vi "IC measurment N6972A - Published.vi"() -> ()   [LabVIEW 2022 SP3]
doc: "This example demonstrates how to configure a list in current priority mode."
uses:
  <vilib>/Analysis/baseanly.llb/Mean (DBL).vi
  <instrlib>/Agilent 34420/Public/Data/Read (Multiple Points).vi
  <instrlib>/Agilent N6900 N7900 Series/Agilent N6900 N7900 Series.lvlib
  <instrlib>/Agilent 34420/Agilent 34420.lvlib
  <vilib>/Analysis/NI_AALBase.lvlib
  <vilib>/Utility/TDMS File Viewer/NI_TDMS File Viewer.lvlib
panel:
  out "Boolean":bool
  out "String":string="WARNING: FILE PATH EXISTS"
  in  "Path":path=path "C:/Users/kumarr3/OneDrive - Victoria University of Wellington - STAFF/Documents/DataFiles/NoLoad" caption="Load File Path or Directory"
  in  "Conduct Experiment\n\n\nLoad Experiment":bool
  in  "relative path (file or folder)":path=path "Test.tdms"
  in  "base path":path=path "C:/Users/kumarr3/OneDrive - Victoria University of Wellington - STAFF/Documents/DataFiles"
  in  "Tab Control":T1(tab)
  in  "N6972A VISA resource name":refnum<visa-resource-name>="USB0::0x0957::0x3407::MY63000447::INSTR"
  in  "Current Priority Voltage Limit":dbl=1.0
  in  "34420A VISA resource name":refnum<visa-resource-name>="COM3"
  in  "Resolution (1E-9)":dbl=1e-09
  in  "Manual Range (0.001)":dbl=0.001
  in  "Auto Range (T: Enable)":bool=TRUE
  in  "Serial Configuration":T2={"Baud Rate"=9600, "Parity"=0, "Data Bits"=8} {"Data Bits" items=["7"=7, "8"=8]; "Parity" items=["None", "Odd", "Even", "Mark", "Space"]; "Baud Rate" items=["300"=300, "600"=600, "1200"=1200, "2400"=2400, "4800"=4800, "9600"=9600]}
  in  "Function (0: DC Volts)":u16(ring) items=["DC Volts", "DC Voltage Ratio", "DC Voltage Difference", "2 Wire Resistance", "4 Wire Resistance", "Temperature"]
  in  "Channel (1: Channel 1)":u16(ring)=1 items=["Channel 1"=1, "Channel 2"=2]
  in  "Filter On/Off":string(combo)
  in  "Voltmeter Offset Sample Count":i32=10
  in  "Integration Time (4: 10 NPLCs)":u16(ring)=4 items=["0.02 NPLC", "0.2 NPLC", "1 NPLC", "2 NPLCs", "10 NPLCs", "20 NPLCs", "100 NPLCs", "200 NPLCs"]
  out "Waveform Chart":dbl(graph)
  in  "Measure Temperature?":bool
  out "Temperature Chart":dbl[](graph)=[25.735546538805686]
  out "?":string
  out "Progress Bar":dbl(slide) scale=0.0..1000.0
  in  "Minutes  / Seconds":bool
  in  "Hours / Minutes":bool
  out "Current Run":i32
  out "Number of Measurements":dbl
  in  "RUN MULTIPLE MEASUREMENTS":bool
  in  "Measurement Interval":dbl
  in  "Total Measurement Time":dbl
  out "XY Graph":cluster{dbl[], dbl[]}(graph)
  out "RMS Current":dbl
  out "uV/cm":dbl
  out "Voltmeter offset (µV)":dbl format="%e"
  out "Current array":dbl[](array[numeric])
  out "Voltage  array":dbl[](array[numeric])
  out "?":bool
  in  "Volt. Tap threshold (uV/cm)":dbl=0.25 format="%.2f"
  in  "Current increment above µV threshold [A]":dbl=0.1 format="%.2f"
  out "?":bool
  in  "Current increment 2 [A]":dbl=0.2 format="%.2f"
  in  "Current limit 1 [A]":dbl=38.0 format="%.2f"
  in  "Initial Current increment  [A]":dbl=5.0 format="%.2f"
  out "Max volt. reached":bool
  out "Max. current reached":bool
  in  "Max. Volt. Tap Voltage (uV/cm)":dbl=10.0
  in  "Maximum current (A)":dbl=48.0
  in  "Volt. Tap Distance (cm)":dbl=1.6
  in  "stop":bool
  out "Calibrating Offset?":bool
  out "Offset V vals":dbl[](array[numeric])
  out "Waiting Time Elapsed":i32 format="%<%H:%M:%S%2u>t"
  out "Start Time":timestamp
  out "Terminated Temp Msre":bool=TRUE
  in  "Temperature Reading Iterval(s)":u32=1
  in  "Ramp interval (s)":u32
  out "median Ic":dbl format="%0.2f"
  out "Current Run":cluster{dbl[], dbl[]}(graph) caption="XY Graph"
  out "Historial Results":cluster{dbl[], dbl[]}[](graph) caption="XY Graph"
  out "Ic Array":dbl[](array[numeric])
  out "n Array":dbl[](array[numeric])
  out "n Values Graph":dbl[](graph)
  out "mean Ic":dbl format="%0.2f"
  out "mean n":dbl format="%0.2f"
  out "Ic Values Graph":dbl[](graph)
  out "median n":dbl format="%0.2f"
  out "Errors?":string[](array[string])
  out "XY Graph 2":cluster{timestamp[], dbl[]}(graph)
  out "median n":dbl format="%0.2f"
  out "n Values Graph":cluster{timestamp[], dbl[]}(graph)
  out "Ic Values Graph":cluster{timestamp[], dbl[]}(graph)
  out "n Array":dbl[](array[numeric])
  out "Ic Array":dbl[](array[numeric])
  out "mean n":dbl format="%0.2f"
  out "mean Ic (A)":dbl format="%0.2f"
  out "Historical Data":cluster{"Array":dbl[], "Array":dbl[]}[](graph)
  out "Number of Runs":dbl
  out "Experiment Description":variant
  out "median Ic (A)":dbl format="%0.2f"
  out "current time":timestamp
  # "Ic Test Controls"
  # "Experiment Control"
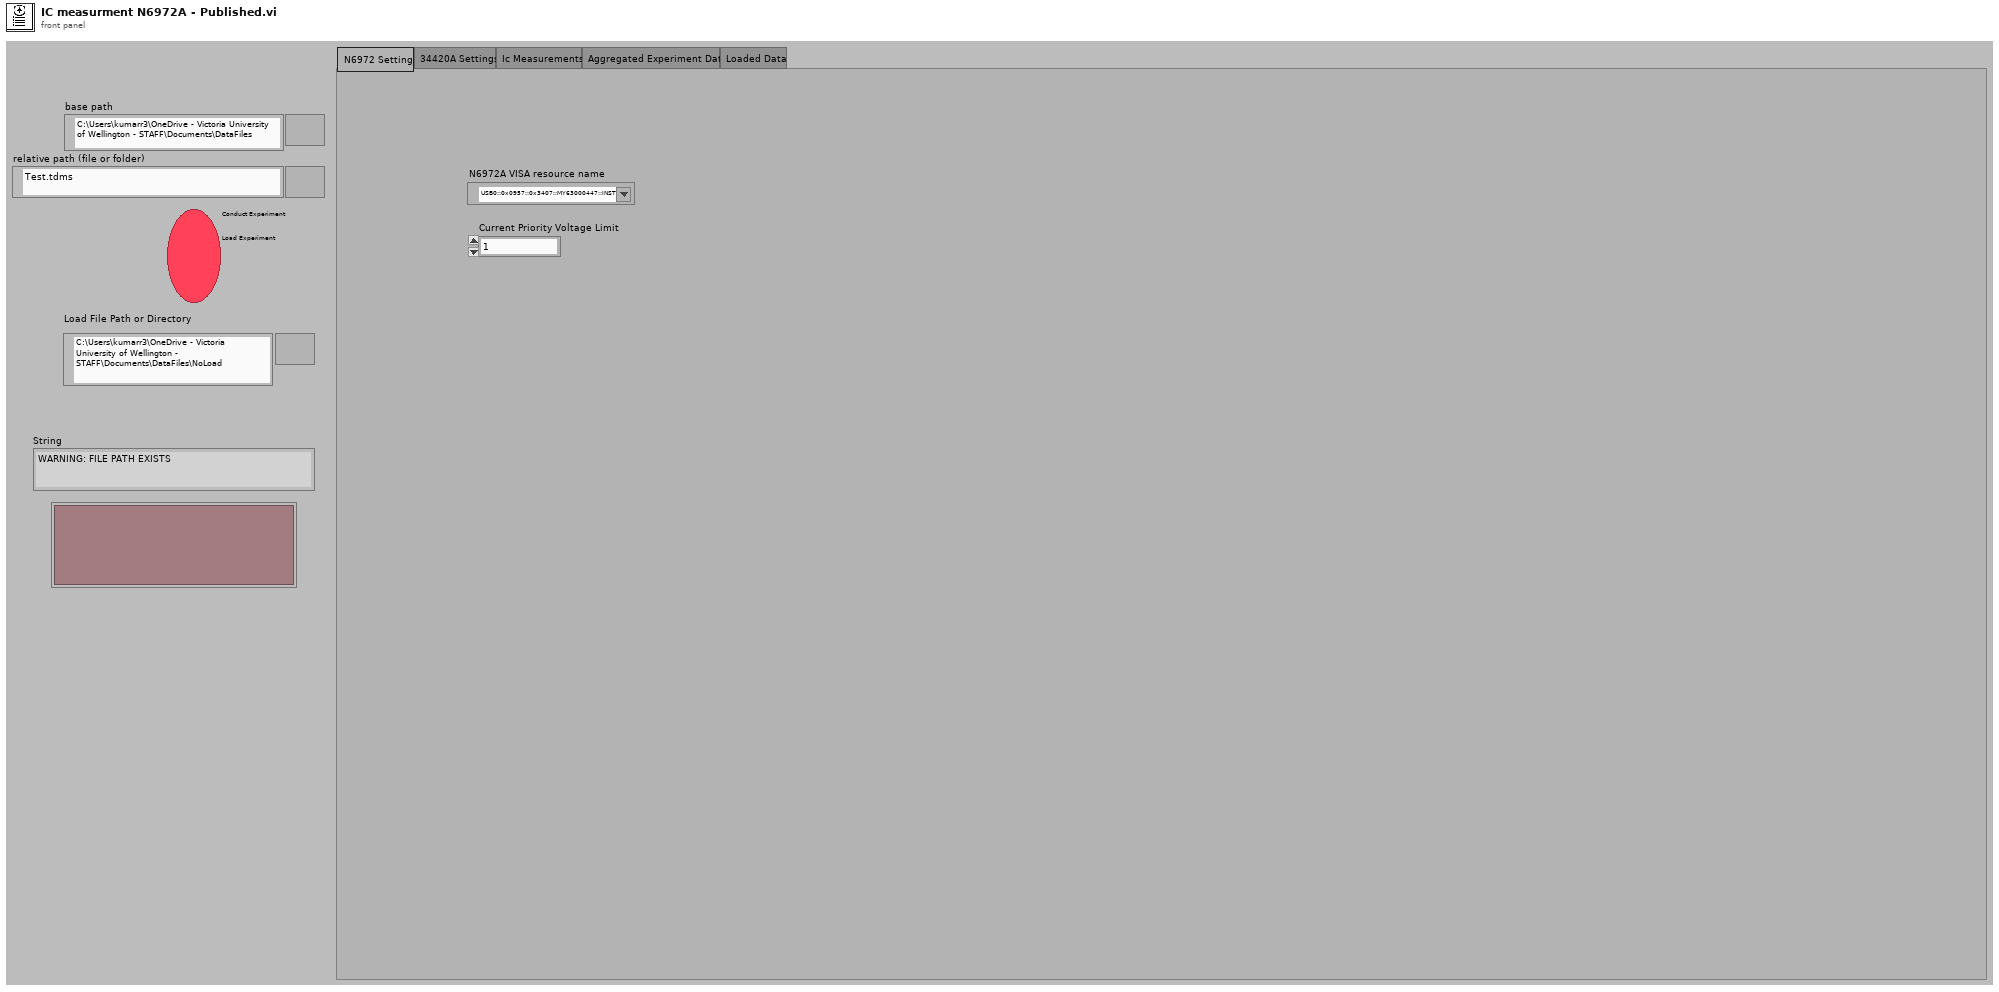
[diagram p1: front panel]
types:
  T1 = enum32{"N6972 Settings", "34420A Settings", "Ic Measurements", "Aggregated Experiment Data", "Loaded Data"}
  T2 = cluster{"Baud Rate":u32, "Parity":u16, "Data Bits":u16}
  T3 = enum16{"open", "open or create", "create or replace", "create", "open (read-only)"}
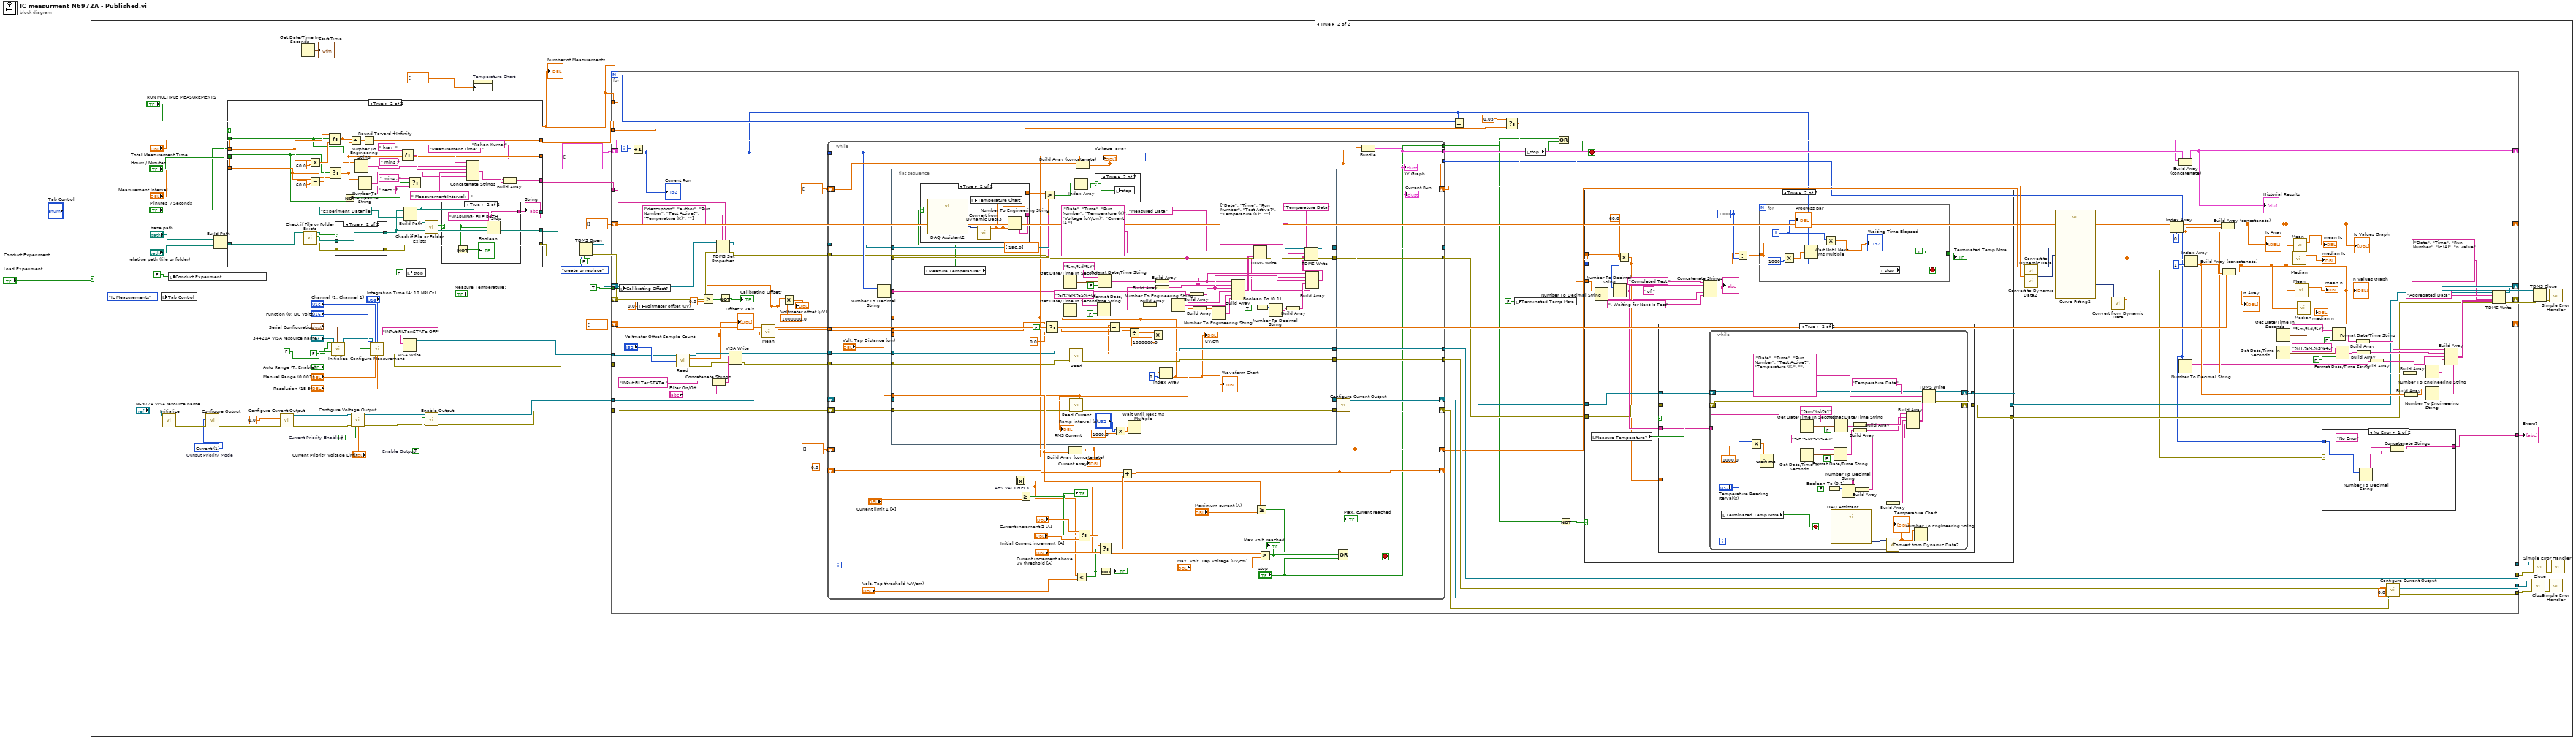
[diagram p0: block diagram]
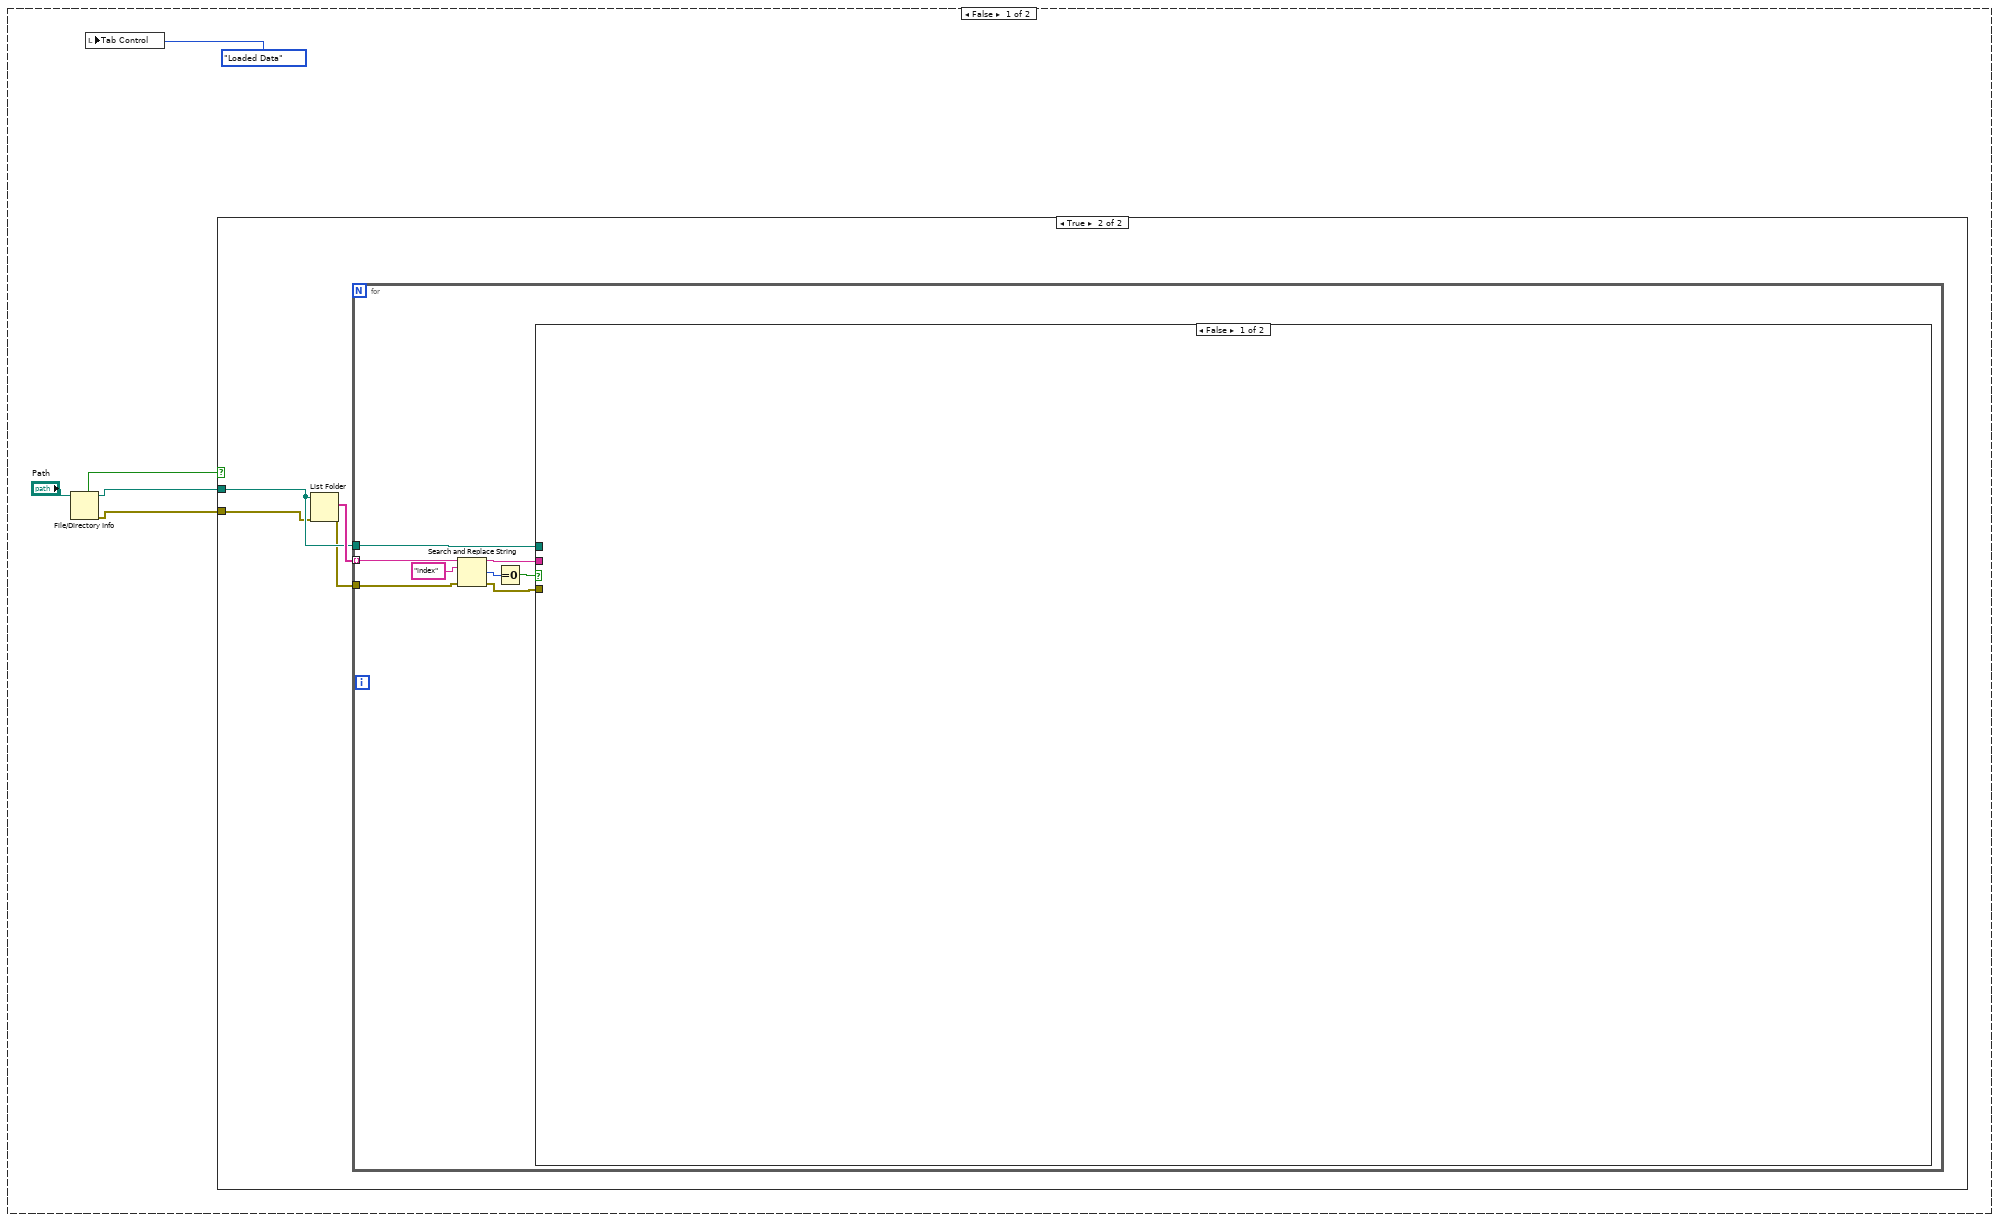
[diagram p2: hidden frame]
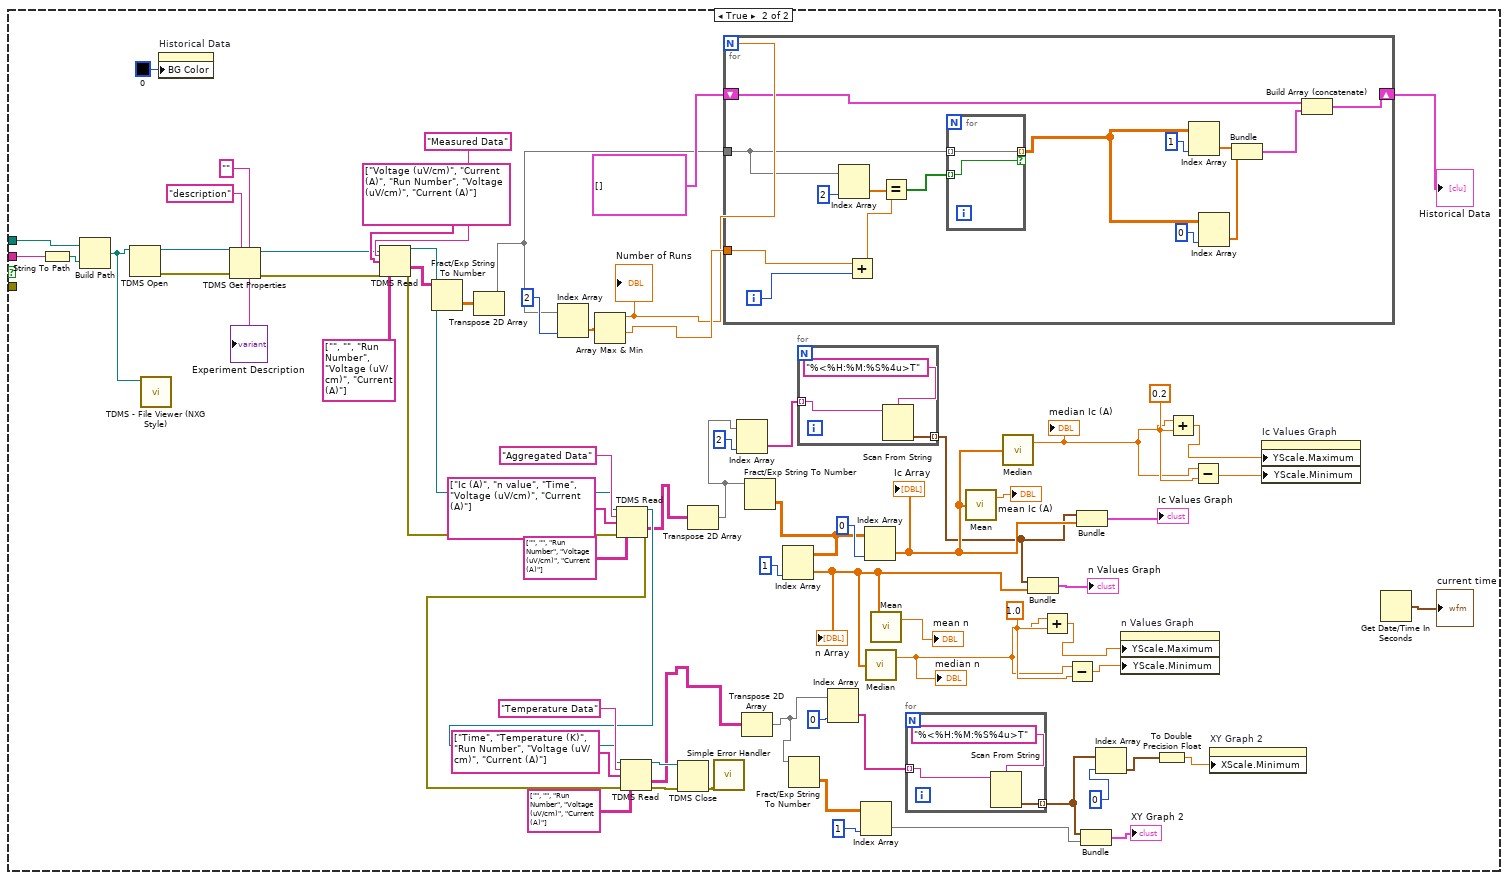
[diagram p4: hidden frame]
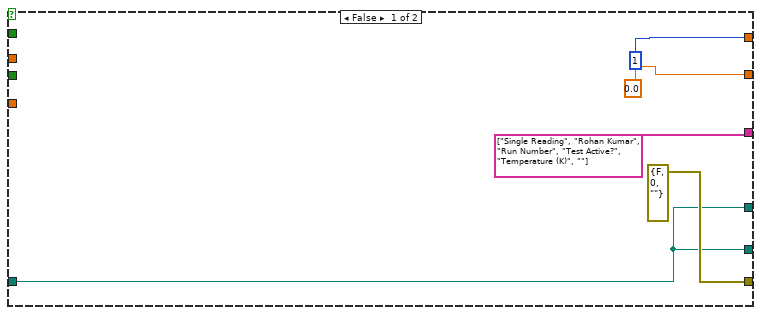
[diagram p5: hidden frame]
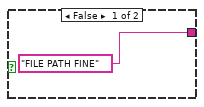
[diagram p6: hidden frame]
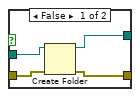
[diagram p7: hidden frame]
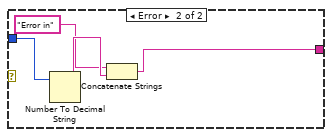
[diagram p8: hidden frame]
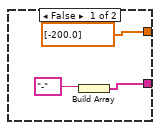
[diagram p12: hidden frame]
diagram:
  n1 = case shown="True" "Conduct Experiment\n\n\nLoad Experiment" {
    frame False {
      n2 = File/Directory Info(path="Path") -> (path out=w5:path, directory=w4:bool, error out=w3:errorcluster)  [unwired: 1 in, 4 out]
      n3 = local write "Tab Control"(T1."Loaded Data" ("Tab Control")) -> ()
      n4 = case shown="True" w4 {
        tunnel: w5 -> [_ w9]
        tunnel: w3 -> [_ w8]
        frame False {
        }
        frame True {
          n5 = List Folder(path=w9, error in=w8) -> (filenames=w10:string[], error out=w7:errorcluster)  [unwired: 2 in, 2 out]
          n6 = for {
            tunnel: w10 -> [w18] mode=indexing
            tunnel: w9 -> [w14]
            tunnel: w7 -> [w12]
            n7 = Search and Replace String(input string=w18, search string="index", error in=w12) -> (result string=w13:string, number of replacements=w16:i32, error out=w11:errorcluster)  [unwired: 5 in, 1 out]
            n8 = Equal To 0?(x=w16) -> (x = 0?=w15:bool)
            n9 = case shown="False" w15 {
              tunnel: w13 -> [_ w90]
              tunnel: w14 -> [_ w89]
              tunnel: w11 -> [_ _]
              frame False {
              }
              frame True {
                w27 = 1.0
                w29 = 0.2
                n10 = String To Path(string=w90) -> (path=w88:path)
                n11 = Build Path(base path=w89, name or relative path=w88) -> (appended path=w19:path)
                n12 = TDMS Open(11:w19) -> (0:w66:errorcluster, 3:w67:refnum<k34>)  [unwired: 6 in]
                n13 = call <vilib>:"TDMS - File Viewer (NXG Style).vi"("file in"=w19) -> ()  [unwired: 9 in, 2 out]
                n14 = property on="Historical Data" class="XYGraph (strict)"("BG Color"=u32 0 ("Plot Area:Colors:BG Color")) -> ()  [unwired: 2 in, 2 out]
                n15 = TDMS Get Properties(5:"", 7:"description", 8:w66, 11:w67) -> (0:w64:errorcluster, 3:w65:refnum<k34>, 4:→"Experiment Description":string)  [unwired: 2 in, 3 out]
                n16 = TDMS Read(0:w65, 5:"Measured Data" ("group name in"), 7:string[] ["Voltage (uV/cm)", "Current (A)", "Run Number", "Voltage (uV/cm)", "Current (A)"] ("channel name(s) in (Untitled)"), 11:w64, 12:string[][] [["", "", "Run Number", "Voltage (uV/cm)", "Current (A)"]] ("channel name(s) in (Untitled)")) -> (4:w54:refnum<k34>, 10:w84:string[][], 15:w53:errorcluster)  [unwired: 3 in, 3 out]
                n17 = Fract/Exp String To Number(string=w84) -> (number=w83:dbl[][])  [unwired: 3 in, 1 out]
                n18 = Transpose 2D Array(2D array=w83) -> (transposed array=w69:dbl[][])
                n19 = Index Array(array=w69, index (col)=2 ("disabled index (col)")) -> (element=w74:dbl[])  [unwired: 1 in]
                n20 = Array Max & Min(array=w74) -> (max value=w72:dbl, min value=w73:dbl)  [unwired: 2 out]
                "Number of Runs" <- w72
                n21 = TDMS Read(0:w54, 5:"Aggregated Data" ("group name in"), 7:string[] ["Ic (A)", "n value", "Time", "Voltage (uV/cm)", "Current (A)"] ("channel name(s) in (Untitled)"), 11:w53, 12:string[][] [["", "", "Run Number", "Voltage (uV/cm)", "Current (A)"]] ("channel name(s) in (Untitled)")) -> (4:w52:refnum<k34>, 10:w34:string[][], 15:w51:errorcluster)  [unwired: 3 in, 3 out]
                n22 = TDMS Read(0:w52, 5:"Temperature Data" ("group name in"), 7:string[] ["Time", "Temperature (K)", "Run Number", "Voltage (uV/cm)", "Current (A)"] ("channel name(s) in (Untitled)"), 11:w51, 12:string[][] [["", "", "Run Number", "Voltage (uV/cm)", "Current (A)"]] ("channel name(s) in (Untitled)")) -> (4:w56:refnum<k34>, 10:w48:string[][], 15:w55:errorcluster)  [unwired: 3 in, 3 out]
                n23 = TDMS Close(8:w55, 11:w56) -> (0:w60:errorcluster)  [unwired: 1 out]
                n24 = Transpose 2D Array(2D array=w34) -> (transposed array=w33:string[][])
                n25 = call <vilib>:"Simple Error Handler.vi"("error in (no error)"=w60) -> ()  [unwired: 2 in, 7 out]
                n26 = for {
                  N: w72 -> [_]
                  tunnel: w69 -> [w105]
                  tunnel: w73 -> [w103]
                  shift-right: [w97] -> w70
                  shift-left: cluster{dbl[], dbl[]}[] [] -> [w99]
                  i -> [w111]
                  n27 = Index Array(array=w105, index (col)=2 ("disabled index (col)")) -> (element=w106:dbl[])  [unwired: 1 in]
                  n28 = Add(x=w103, y=w111) -> (x+y=w104:dbl)
                  n29 = Equal?(x=w106, y=w104) -> (x = y?=w101:bool[])
                  n30 = for {
                    tunnel: w101 -> [w112] mode=indexing
                    tunnel: w105 -> [w113] mode=indexing
                    tunnel: [w113] -> w102 mode=indexing if=w112
                  }
                  n31 = Index Array(array=w102, index (col)=1 ("disabled index (col)")) -> (element=w108:dbl[])  [unwired: 1 in]
                  n32 = Index Array(array=w102, index (col)=0 ("disabled index (col)")) -> (element=w107:dbl[])  [unwired: 1 in]
                  n33 = Bundle(w108, w107) -> (w98:cluster{dbl[], dbl[]})  [unwired: 1 in]
                  n34 = Build Array (concatenate)(w99, w98) -> (w97:cluster{dbl[], dbl[]}[])
                }
                "Historical Data" <- w70
                n35 = Index Array(array=w33, index (col)=2 ("disabled index (col)")) -> (element=w40:string[])  [unwired: 1 in]
                n36 = Transpose 2D Array(2D array=w48) -> (transposed array=w45:string[][])
                n37 = Fract/Exp String To Number(string=w33) -> (number=w32:dbl[][])  [unwired: 3 in, 1 out]
                n38 = Index Array(array=w32, index (col)=1 ("disabled index (col)")) -> (element=w39:dbl[])  [unwired: 1 in]
                "n Array" <- w39
                n39 = Fract/Exp String To Number(string=w45) -> (number=w47:dbl[][])  [unwired: 3 in, 1 out]
                n40 = for {
                  tunnel: w40 -> [w93] mode=indexing
                  tunnel: [w91] -> w36 mode=indexing
                  n41 = Scan From String(format string="%<%H:%M:%S%4u>T" ("time format string (%c)"), input string=w93) -> (output 1=w91:timestamp)  [unwired: 3 in, 3 out]
                }
                n42 = Index Array(array=w45, index (col)=0 ("disabled index (col)")) -> (element=w44:string[])  [unwired: 1 in]
                n43 = Index Array(array=w47, index (col)=1 ("disabled index (col)")) -> (element=w43:dbl[])  [unwired: 1 in]
                n44 = Index Array(array=w32, index (col)=0 ("disabled index (col)")) -> (element=w37:dbl[])  [unwired: 1 in]
                "Ic Array" <- w37
                n45 = call <vilib>:"Median.vi"("X"=w39) -> ("median"=w24:dbl)  [unwired: 1 out]
                "median n" <- w24
                n46 = call-poly <vilib>:"Mean.vi"("X"=w39) -> ("mean"=→"mean n":dbl)  [unwired: 1 out]
                n47 = for {
                  tunnel: w44 -> [w96] mode=indexing
                  tunnel: [w94] -> w23 mode=indexing
                  n48 = Scan From String(format string="%<%H:%M:%S%4u>T" ("time format string (%c)"), input string=w96) -> (output 1=w94:timestamp)  [unwired: 3 in, 3 out]
                }
                n49 = call-poly <vilib>:"Mean.vi"("X"=w37) -> ("mean"=→"mean Ic (A)":dbl)  [unwired: 1 out]
                n50 = call <vilib>:"Median.vi"("X"=w37) -> ("median"=w28:dbl)  [unwired: 1 out]
                "median Ic (A)" <- w28
                n51 = Bundle(w36, w39) -> (→"n Values Graph":cluster{timestamp[], dbl[]})  [unwired: 1 in]
                n52 = Add(x=w24, y=w27) -> (x+y=w26:dbl)
                n53 = Subtract(x=w24, y=w27) -> (x-y=w25:dbl)
                n54 = Bundle(w36, w37) -> (→"Ic Values Graph":cluster{timestamp[], dbl[]})  [unwired: 1 in]
                n55 = Bundle(w23, w43) -> (→"XY Graph 2":cluster{timestamp[], dbl[]})  [unwired: 1 in]
                n56 = Index Array(array=w23, index=0 ("disabled index (col)")) -> (element=w21:timestamp)
                n57 = property on="n Values Graph" class="XYGraph (strict)"("YScale.Maximum"=w26, "YScale.Minimum"=w25) -> ()  [unwired: 2 in, 2 out]
                n58 = To Double Precision Float(number=w21) -> (double precision float=w20:dbl)
                n59 = Add(x=w28, y=w29) -> (x+y=w30:dbl)
                n60 = Subtract(x=w28, y=w29) -> (x-y=w31:dbl)
                n61 = property on="XY Graph 2" class="XYGraph (strict)"("XScale.Minimum"=w20) -> ()  [unwired: 2 in, 2 out]
                n62 = property on="Ic Values Graph" class="XYGraph (strict)"("YScale.Maximum"=w30, "YScale.Minimum"=w31) -> ()  [unwired: 2 in, 2 out]
                n63 = Get Date/Time In Seconds() -> (seconds since 1Jan1904=→"current time":timestamp)
              }
            }
          }
        }
      }
    }
    frame True {
      w175 = TRUE  # Enable Output
      w172 = TRUE  # Current Priority Enabled
      w179 = u16 1 items=["Voltage", "Current"]  # Output Priority Mode
      n64 = local write "Tab Control"(T1."Ic Measurements" ("Tab Control")) -> ()
      n65 = call <instrlib>:"Initialize.vi"("VISA resource name"="N6972A VISA resource name") -> ("error out"=w180:errorcluster, "VISA resource name out"=w181:refnum<visa-resource-name>)  [unwired: 9 in]
      n66 = local write "Conduct Experiment\n\n\nLoad Experiment"(FALSE) -> ()
      n67 = call <instrlib>:"Configure Output.vi"("error in (no error)"=w180, "Output Priority Mode (0: Voltage)"=w179, "VISA resource name"=w181) -> ("error out"=w177:errorcluster, "VISA resource name out"=w178:refnum<visa-resource-name>)  [unwired: 7 in]
      n68 = Build Path(base path="base path", name or relative path="relative path (file or folder)") -> (appended path=w134:path)
      n69 = case shown="True" "RUN MULTIPLE MEASUREMENTS" {
        tunnel: "Total Measurement Time" -> [_ w213]
        tunnel: "Measurement Interval" -> [_ w210]
        tunnel: [u8 1 w221] -> w119
        tunnel: [0.0 ("Measurement Interval (Minutes)") w199] -> w133
        tunnel: w134 -> [w183 w219]
        tunnel: [w183 w193] -> w128
        tunnel: [errorcluster {"status"=FALSE, "code"=0, "source"=""} ("error out") w216] -> w130
        tunnel: "Hours / Minutes" -> [_ w200]
        tunnel: "Minutes  / Seconds" -> [_ w189]
        tunnel: [w183 w209] -> _
        tunnel: [string[] ["Single Reading", "Rohan Kumar", "Run Number", "Test Active?", "Temperature (K)", ""] ("channel name(s) in (Untitled)") w194] -> w120
        frame False {
        }
        frame True {
          n70 = call <vilib>:"Check if File or Folder Exists.vi"("path"=w219) -> ("error out"=w217:errorcluster, "file or folder exists?"=w218:bool, "dup path"=w215:path)  [unwired: 8 in]
          n71 = Multiply(x=w213, y=60.0) -> (x*y=w212:dbl)
          n72 = Divide(x=w210, y=60.0) -> (x/y=w211:dbl)
          n73 = Select(t=w213, s=w200, f=w212) -> (s? t:f=w187:dbl)
          n74 = Select(t=w211, s=w189, f=w210) -> (s? t:f=w199:dbl)
          n75 = case shown="True" w218 {
            tunnel: w217 -> [w230 w231]
            tunnel: [w229 w231] -> w216
            tunnel: [w228 w232] -> w209
            tunnel: w215 -> [w227 w232]
            frame False {
              n76 = Create Folder(path (use dialog)=w227, error in=w230) -> (created path=w228:path, error out=w229:errorcluster)  [unwired: 1 in, 1 out]
            }
            frame True {
            }
          }
          n77 = Not(x=w189) -> (.not. x?=w188:bool)
          n78 = Divide(x=w187, y=w199) -> (x/y=w190:dbl)
          n79 = Number To Engineering String(4:w187) -> (0:w197:string)  [unwired: 3 in]
          n80 = Number To Engineering String(4:w199) -> (0:w198:string)  [unwired: 3 in]
          n81 = Round Toward +Infinity(x=w190) -> (ceil(x): smallest int >= x=w221:dbl)
          n82 = Select(t=" hrs ;  ", s=w200, f=" mins ;") -> (s? t:f=w203:string)
          n83 = Build Path(base path=w209, name or relative path=path "Experiment_DataFile") -> (appended path=w193:path)
          n84 = Select(t=" mins ; ", s=w188, f=" secs ; ") -> (s? t:f=w201:string)
          n85 = call <vilib>:"Check if File or Folder Exists.vi"("path"=w193) -> ("file or folder exists?"=w192:bool)  [unwired: 8 in, 2 out]
          n86 = case shown="True" w192 {
            selector: w192 -> [_ w225]
            tunnel: ["FILE PATH FINE" "WARNING: FILE PATH EXISTS"] -> w191
            frame False {
            }
            frame True {
              n87 = Not(x=w225) -> (.not. x?=→"Boolean":bool)
              n88 = Stop(stop? (T)=w225) -> ()
            }
          }
          "String" <- w191
          n89 = Concatenate Strings("Measurement Time:   ", w197, w203, " Measurement Interval:   ", w198, w201) -> (w195:string)
          n90 = Build Array(w195, "Rohan Kumar") -> (w194:string[])
        }
      }
      "Number of Measurements" <- w119
      n91 = call <instrlib>:"Configure Current Output.vi"("VISA resource name"=w178, "Current Immediate Amplitude (0 A)"=0.0, "error in (no error)"=w177) -> ("VISA resource name out"=w173:refnum<visa-resource-name>, "error out"=w174:errorcluster)  [unwired: 11 in]
      n92 = Get Date/Time In Seconds() -> (seconds since 1Jan1904=→"Start Time":timestamp)
      n93 = call <instrlib>:"Initialize.vi"("Serial Configuration"="Serial Configuration", "Reset (True)"=FALSE, "ID Query (True)"=FALSE, "VISA resource name"="34420A VISA resource name") -> ("error out"=w163:errorcluster, "VISA resource name out"=w162:refnum<visa-resource-name>)  [unwired: 6 in]
      n94 = call <instrlib>:"Configure Voltage Output.vi"("VISA resource name"=w173, "error in (no error)"=w174, "Enable Current Priority (False)"=w172, "Current Priority Voltage Limit (25V)"="Current Priority Voltage Limit") -> ("VISA resource name out"=w170:refnum<visa-resource-name>, "error out"=w169:errorcluster)  [unwired: 10 in]
      n95 = call <instrlib>:"Configure Measurement.vi"("VISA resource name"=w162, "Channel (1: Channel 1)"="Channel (1: Channel 1)", "Integration Time (4: 10 NPLCs)"="Integration Time (4: 10 NPLCs)", "Function (0: DC Volts)"="Function (0: DC Volts)", "Auto Range (T:Enable)"="Auto Range (T: Enable)", "error in (no error)"=w163, "Manual Range (0.001)"="Manual Range (0.001)", "Resolution (1E-9)"="Resolution (1E-9)") -> ("VISA resource name out"=w157:refnum<visa-resource-name>, "error out"=w150:errorcluster)  [unwired: 6 in]
      n96 = VISA Write(VISA resource name=w157, write buffer="INPut:FILTer:STATe OFF") -> (VISA resource name out=w151:refnum<visa-resource-name>)  [unwired: 1 in, 2 out]
      n97 = local write "stop"(FALSE ("stop")) -> ()
      n98 = call <instrlib>:"Enable Output.vi"("error in (no error)"=w169, "Enable Output (F: Disable)"=w175, "VISA resource name"=w170) -> ("error out"=w154:errorcluster, "VISA resource name out"=w155:refnum<visa-resource-name>)  [unwired: 7 in]
      n99 = property on="Temperature Chart" class="WFChart (strict)"("History Data"=dbl[] []) -> ()  [unwired: 2 in, 2 out]
      n100 = TDMS Open(6:FALSE ("disable buffering (T)"), 8:w130, 10:T3."create or replace" ("operation"), 11:w128) -> (0:w127:errorcluster, 3:w126:refnum<k34>)  [unwired: 3 in]
      n101 = for {
        N: w119 -> [w266]
        tunnel: w155 -> [w325]
        tunnel: w154 -> [w324]
        tunnel: w133 -> [w263]
        tunnel: w151 -> [w315]
        tunnel: w150 -> [w314]
        tunnel: [w311] -> w148
        tunnel: [w310] -> w147
        tunnel: [w309] -> w145
        tunnel: [w278] -> w144
        shift-right: [w298] -> _
        shift-left: cluster{dbl[], dbl[]}[] [] -> [w306]
        shift-right: [w244] -> _
        shift-left: dbl[] [] -> [w302]
        shift-right: [w247] -> _
        shift-left: dbl[] [] -> [w299]
        shift-right: [w272] -> w125
        shift-left: w126 -> [w254]
        shift-right: [w273] -> w132
        shift-left: w127 -> [w253]
        tunnel: TRUE ("x > y?") -> [w258]
        tunnel: w120 -> [w249]
        tunnel: w119 -> [w248]
        tunnel: [w235] -> w115 mode=indexing
        i -> [w308]
        stop <- w256 stop-if-true
        n102 = local write "Calibrating Offset?"(w258) -> ()
        n103 = Increment(x=w308) -> (x+1=w265:i32)
        "Current Run" <- w265
        n104 = local write "Voltmeter offset (µV)"(0.0 ("Voltmeter offset (v)")) -> ()
        n105 = call-poly <instrlib>:"Read.vi"("VISA resource name"=w315, "Sample Count (1)"="Voltmeter Offset Sample Count", "error in (no error)"=w314) -> ("VISA resource name out"=w321:refnum<visa-resource-name>, "Measurements"=w243:dbl[], "error out"=w322:errorcluster)  [unwired: 10 in]
        "Offset V vals" <- w243
        n106 = Concatenate Strings("INPut:FILTer:STATe ", "Filter On/Off") -> (w323:string)
        n107 = TDMS Set Properties(5:w249, 7:string[] ["description", "author", "Run Number", "Test Active?", "Temperature (K)", ""] ("channel name(s) in (Untitled)"), 8:w253, 11:w254) -> (0:w252:errorcluster, 3:w251:refnum<k34>)  [unwired: 2 in, 2 out]
        n108 = VISA Write(VISA resource name=w321, write buffer=w323, error in (no error)=w322) -> (VISA resource name out=w312:refnum<visa-resource-name>, error out=w313:errorcluster)  [unwired: 1 out]
        n109 = call-poly <vilib>:"Mean.vi"("X"=w243) -> ("mean"=w242:dbl)  [unwired: 1 out]
        n110 = Greater?(x=w242, y=0.0) -> (0:w259:bool)
        n111 = Not(x=w259) -> (.not. x?=→"Calibrating Offset?":bool)
        n112 = Multiply(x=w242, y=1000000.0) -> (x*y=→"Voltmeter offset (µV)":dbl)
        n113 = while {
          shift-right: [w434] -> w330
          shift-left: w325 -> [w447]
          shift-right: [w432] -> w329
          shift-left: w324 -> [w427]
          shift-right: [w431] -> _
          shift-left: 0.0 -> [w436]
          shift-right: [w416] -> w304
          shift-left: dbl[] [] -> [w430]
          tunnel: [w429] -> w309
          tunnel: [w428] -> w278
          shift-right: [w415] -> w305
          shift-left: dbl[] [] -> [w426]
          tunnel: w312 -> [w419]
          tunnel: w313 -> [w418]
          tunnel: w242 -> [w417]
          tunnel: [w414] -> w270
          tunnel: [w413] -> w269
          tunnel: ["stop"] -> w257
          tunnel: [w406] -> w307
          tunnel: [w410] -> w234
          tunnel: w265 -> [w410]
          tunnel: w252 -> [w408]
          tunnel: w251 -> [w407]
          stop <- w412 stop-if-true
          n114 = Number To Decimal String(number=w410) -> (decimal integer string=w409:string)  [unwired: 1 in]
          n115 = flat-sequence {
            tunnel: w447 -> [w509]
            tunnel: w427 -> [w508]
            tunnel: [w507] -> w435
            tunnel: [w506] -> w433
            tunnel: [w482] -> w421
            tunnel: [w505] -> w429
            tunnel: [w504] -> w428
            tunnel: [w459] -> w405
            tunnel: "Volt. Tap Distance (cm)" -> [w503]
            tunnel: w419 -> [w499]
            tunnel: w418 -> [w498]
            tunnel: w417 -> [w453]
            tunnel: w407 -> [w495]
            tunnel: [w476] -> w414
            tunnel: w408 -> [w494]
            tunnel: [w473] -> w413
            tunnel: w409 -> [w481]
            frame #0 {
              n116 = local read "Measure Temperature?"() -> (w461:bool)
              n117 = case shown="True" w461 {
                tunnel: [w512 w515] -> w462
                tunnel: [dbl[] [-200.0] ("Array") w514] -> w458
                frame False {
                  n118 = Build Array("-" ("group name")) -> (w512:string[])
                }
                frame True {
                  n119 = call "DAQ Assistant2"() -> ("data"=w516:dynamicdata)  [unwired: 17 in, 2 out]
                  n120 = call "Convert from Dynamic Data3"("Dynamic Data Type"=w516) -> ("Array"=w514:dbl[])  [unwired: 3 in]
                  n121 = local write "Temperature Chart"(w514) -> ()
                  n122 = Number To Engineering String(4:w514) -> (0:w515:string[])  [unwired: 3 in]
                }
              }
              n123 = Greater Or Equal?(x=w458, y=dbl[] [-196.0]) -> (x >= y?=w455:bool[])
              n124 = Select(t=w453, s=FALSE, f=0.0) -> (s? t:f=w452:dbl)
              n125 = Get Date/Time In Seconds() -> (seconds since 1Jan1904=w488:timestamp)
              n126 = Get Date/Time In Seconds() -> (seconds since 1Jan1904=w491:timestamp)
              n127 = call-poly <instrlib>:"Read.vi"("VISA resource name"=w499, "error in (no error)"=w498) -> ("VISA resource name out"=w504:refnum<visa-resource-name>, "Measurements"=w460:dbl[], "error out"=w505:errorcluster)  [unwired: 11 in]
              n128 = call <instrlib>:"Read Current.vi"("VISA resource name"=w509, "error in (no error)"=w508) -> ("RMS Current"=w482:dbl, "VISA resource name out"=w507:refnum<visa-resource-name>, "error out"=w506:errorcluster)  [unwired: 6 in, 5 out]
              "RMS Current" <- w482
              n129 = Index Array(array=w455) -> (element=w456:bool)  [unwired: 1 in]
              n130 = case shown="True" w456 {
                selector: w456 -> [_ w510]
                frame False {
                }
                frame True {
                  n131 = local write "stop"(w510) -> ()
                }
              }
              n132 = Format Date/Time String(time format string (%c)="%H:%M:%S%4u", seconds (now)=w491, UTC format=FALSE) -> (date/time string=w486:string)
              n133 = Format Date/Time String(time format string (%c)="%m/%d/%Y", seconds (now)=w488, UTC format=FALSE) -> (date/time string=w487:string)
              n134 = Subtract(x=w460, y=w452) -> (x-y=w500:dbl[])
              n135 = Multiply(x="Ramp interval (s)", y=1000.0) -> (x*y=w449:dbl)
              n136 = Divide(x=w500, y=w503) -> (x/y=w502:dbl[])
              n137 = Wait Until Next ms Multiple(millisecond multiple=w449) -> ()  [unwired: 1 out]
              n138 = Multiply(x=w502, y=1000000.0) -> (x*y=w479:dbl[])
              n139 = Build Array(w487) -> (w464:string[])
              n140 = Build Array(w486) -> (w463:string[])
              n141 = Index Array(array=w479, index=0) -> (element=w459:dbl)
              "uV/cm" <- w459
              "Waveform Chart" <- w459
              n142 = Build Array(w459) -> (w485:dbl[])
              n143 = Number To Engineering String(4:w485) -> (0:w478:string[])  [unwired: 3 in]
              n144 = Build Array(w481) -> (w465:string[])
              n145 = Build Array(w482) -> (w483:dbl[])
              n146 = Number To Engineering String(4:w483) -> (0:w477:string[])  [unwired: 3 in]
              n147 = Build Array(w464, w463, w465, w462, w478, w477) -> (w484:string[][])
              n148 = TDMS Write(0:w495, 5:"Measured Data" ("group name"), 7:string[] ["Date", "Time", "Run Number", "Temperature (K)", "Voltage (uV/cm)", "Current (A)"] ("channel name(s) in (Untitled)"), 9:w484, 11:w494) -> (4:w475:refnum<k34>, 15:w474:errorcluster)  [unwired: 1 in, 2 out]
              n149 = Boolean To (0,1)(Boolean=TRUE) -> (0, 1=w469:i16)
              n150 = Number To Decimal String(number=w469) -> (decimal integer string=w466:string)  [unwired: 1 in]
              n151 = Build Array(w466) -> (w467:string[])
              n152 = Build Array(w464, w463, w465, w467, w462) -> (w468:string[][])
              n153 = TDMS Write(0:w475, 5:"Temperature Data" ("group name"), 7:string[] ["Date", "Time", "Run Number", "Test Active?", "Temperature (K)", ""] ("channel name(s) in (Untitled)"), 9:w468, 11:w474) -> (4:w476:refnum<k34>, 15:w473:errorcluster)  [unwired: 1 in, 2 out]
            }
          }
          n154 = Absolute Value "ABS VAL CHECK"(x=w405) -> (abs(x)=w404:dbl)
          n155 = Greater Or Equal?(x=w421, y="Current limit 1 [A]") -> (x >= y?=w438:bool)
          "?" <- w438
          n156 = Build Array (concatenate)(w430, w421) -> (w416:dbl[])
          "Current array" <- w416
          n157 = Less?(x=w404, y="Volt. Tap threshold (uV/cm)") -> (x < y?=w440:bool)
          n158 = Build Array (concatenate)(w426, w405) -> (w415:dbl[])
          "Voltage  array" <- w415
          n159 = Select(t="Current increment 2 [A]", s=w438, f="Initial Current increment  [A]") -> (s? t:f=w442:dbl)
          n160 = Select(t=w442, s=w440, f="Current increment above µV threshold [A]") -> (s? t:f=w437:dbl)
          n161 = Not(x=w440) -> (.not. x?=→"?":bool)
          n162 = Add(x=w436, y=w437) -> (x+y=w431:dbl)
          n163 = Greater Or Equal?(x=w421, y="Maximum current (A)") -> (x >= y?=w424:bool)
          "Max. current reached" <- w424
          n164 = Greater Or Equal?(x=w404, y="Max. Volt. Tap Voltage (uV/cm)") -> (x >= y?=w422:bool)
          "Max volt. reached" <- w422
          n165 = call <instrlib>:"Configure Current Output.vi"("VISA resource name"=w435, "Current Immediate Amplitude (0 A)"=w431, "error in (no error)"=w433) -> ("VISA resource name out"=w434:refnum<visa-resource-name>, "error out"=w432:errorcluster)  [unwired: 11 in]
          n166 = Compound Arithmetic op=OR(w424, w422, "stop") -> (w412:bool)
          n167 = Bundle(w416, w415) -> (w406:cluster{dbl[], dbl[]})  [unwired: 1 in]
          "XY Graph" <- w406
          "Current Run" <- w406
        }
        n168 = Equal?(x=w266, y=w265) -> (x = y?=w264:bool)
        n169 = Select(t=0.05, s=w264, f=w263) -> (s? t:f=w262:dbl)
        n170 = local write "Terminated Temp Msre"(FALSE ("Terminated Temp Msre")) -> ()
        n171 = local read "stop"() -> (w255:bool)
        n172 = Compound Arithmetic op=OR(w257, w255) -> (w256:bool)
        n173 = Not(x=w257) -> (.not. x?=w277:bool)
        n174 = case shown="True" w277 {
          tunnel: w265 -> [_ w359]
          tunnel: w270 -> [w341 w353]
          tunnel: w269 -> [w340 w352]
          tunnel: [w341 w351] -> w268
          tunnel: [w340 w350] -> w267
          tunnel: w262 -> [_ w349]
          tunnel: w248 -> [_ w344]
          frame False {
          }
          frame True {
            w357 = 1000
            n175 = local read "Measure Temperature?"() -> (w347:bool)
            n176 = Number To Decimal String(number=w344) -> (decimal integer string=w343:string)  [unwired: 1 in]
            n177 = Number To Decimal String(number=w359) -> (decimal integer string=w354:string)  [unwired: 1 in]
            n178 = Multiply(x=w349, y=60.0) -> (x*y=w348:dbl)
            n179 = case shown="True" w347 {
              tunnel: w354 -> [_ w367]
              tunnel: w353 -> [w362 w366]
              tunnel: w352 -> [w361 w365]
              tunnel: [w362 w364] -> w351
              tunnel: [w361 w363] -> w350
              tunnel: w348 -> [_ _]
              frame False {
              }
              frame True {
                n180 = while {
                  tunnel: w367 -> [w384]
                  shift-right: [w380] -> w364
                  shift-left: w366 -> [w382]
                  shift-right: [w379] -> w363
                  shift-left: w365 -> [w381]
                  stop <- w368 stop-if-true
                  (unwired) FALSE ("UTC format")
                  n181 = local read "Terminated Temp Msre"() -> (w368:bool)
                  n182 = Multiply(x="Temperature Reading Iterval(s)", y=1000.0) -> (x*y=w376:dbl)
                  n183 = Wait (ms)(milliseconds to wait=w376) -> ()  [unwired: 1 out]
                  n184 = Get Date/Time In Seconds() -> (seconds since 1Jan1904=w390:timestamp)
                  n185 = Get Date/Time In Seconds() -> (seconds since 1Jan1904=w393:timestamp)
                  n186 = Boolean To (0,1)(Boolean=FALSE) -> (0, 1=w372:i16)
                  n187 = call "DAQ Assistant"() -> ("data"=w383:dynamicdata)  [unwired: 17 in, 2 out]
                  n188 = Format Date/Time String(time format string (%c)="%H:%M:%S%4u", seconds (now)=w393) -> (date/time string=w388:string)  [unwired: 1 in]
                  n189 = Format Date/Time String(time format string (%c)="%m/%d/%Y", seconds (now)=w390, UTC format=FALSE) -> (date/time string=w389:string)
                  n190 = Number To Decimal String(number=w372) -> (decimal integer string=w370:string)  [unwired: 1 in]
                  n191 = Build Array(w389) -> (w387:string[])
                  n192 = Build Array(w388) -> (w386:string[])
                  n193 = Build Array(w370) -> (w369:string[])
                  n194 = call "Convert from Dynamic Data2"("Dynamic Data Type"=w383) -> ("Array"=w375:dbl[])  [unwired: 3 in]
                  "Temperature Chart" <- w375
                  n195 = Build Array(w384) -> (w371:string[])
                  n196 = Number To Engineering String(4:w375) -> (0:w374:string[])  [unwired: 3 in]
                  n197 = Build Array(w387, w386, w371, w369, w374) -> (w385:string[][])
                  n198 = TDMS Write(0:w382, 5:"Temperature Data" ("group name"), 7:string[] ["Date", "Time", "Run Number", "Test Active?", "Temperature (K)", ""] ("channel name(s) in (Untitled)"), 9:w385, 11:w381) -> (4:w380:refnum<k34>, 15:w379:errorcluster)  [unwired: 1 in, 2 out]
                }
              }
            }
            n199 = Concatenate Strings("Completed Test ", w354, " of " ("Title"), w343, ". Waiting for Next Ic Test" ("Title")) -> (→"?":string)
            n200 = Divide(x=w348, y=w357) -> (x/y=w356:dbl)
            n201 = for {
              N: w357 -> [_]
              tunnel: w356 -> [w400]
              tunnel: [TRUE] -> w342
              i -> [w401]
              stop <- w398 stop-if-true
              n202 = Multiply(x=w400, y=u32 1000 ("millisecond multiple")) -> (x*y=w402:dbl)
              n203 = Wait Until Next ms Multiple(millisecond multiple=w402) -> ()  [unwired: 1 out]
              n204 = Multiply(x=w401, y=w400) -> (x*y=→"Waiting Time Elapsed":dbl)
              n205 = local read "stop"() -> (w398:bool)
              "Progress Bar" <- w401
            }
            "Terminated Temp Msre" <- w342
          }
        }
        n206 = call "Convert to Dynamic Data"("Array"=w304) -> ("Dynamic Data Type"=w238:dynamicdata)  [unwired: 3 in]
        n207 = call "Convert to Dynamic Data2"("Array"=w305) -> ("Dynamic Data Type"=w239:dynamicdata)  [unwired: 3 in]
        n208 = call "Curve Fitting2"("Locations"=w238, "Signals"=w239) -> ("error out"=w236:errorcluster, "non-linear coefficients"=w237:dynamicdata)  [unwired: 5 in, 3 out]
        n209 = call "Convert from Dynamic Data"("Dynamic Data Type"=w237) -> ("Array"=w301:dbl[])  [unwired: 3 in]
        n210 = Index Array(array=w301, index=0) -> (element=w276:dbl)
        n211 = Build Array (concatenate)(w306, w307) -> (w298:cluster{dbl[], dbl[]}[])
        "Historial Results" <- w298
        n212 = Number To Decimal String(number=w234) -> (decimal integer string=w275:string)  [unwired: 1 in]
        n213 = Index Array(array=w301, index=1) -> (element=w280:dbl)
        n214 = Build Array (concatenate)(w302, w276) -> (w244:dbl[])
        "Ic Array" <- w244
        "Ic Values Graph" <- w244
        n215 = Build Array (concatenate)(w299, w280) -> (w247:dbl[])
        "n Values Graph" <- w247
        "n Array" <- w247
        n216 = Get Date/Time In Seconds() -> (seconds since 1Jan1904=w290:timestamp)
        n217 = Get Date/Time In Seconds() -> (seconds since 1Jan1904=w293:timestamp)
        n218 = call <vilib>:"Median.vi"("X"=w244) -> ("median"=→"median Ic":dbl)  [unwired: 1 out]
        n219 = call-poly <vilib>:"Mean.vi"("X"=w244) -> ("mean"=→"mean Ic":dbl)  [unwired: 1 out]
        n220 = call-poly <vilib>:"Mean.vi"("X"=w247) -> ("mean"=→"mean n":dbl)  [unwired: 1 out]
        n221 = call <vilib>:"Median.vi"("X"=w247) -> ("median"=→"median n":dbl)  [unwired: 1 out]
        n222 = case shown="No Error" w236 {
          tunnel: [w332 w339] -> w235
          tunnel: w234 -> [w334 w336]
          frame No Error {
            n223 = Number To Decimal String(number=w334) -> (decimal integer string=w335:string)  [unwired: 1 in]
            n224 = Concatenate Strings("No Error" ("group name in"), w335) -> (w332:string)
          }
          frame Error {
            n225 = Number To Decimal String(number=w336) -> (decimal integer string=w338:string)  [unwired: 1 in]
            n226 = Concatenate Strings("Error in" ("group name in"), w338) -> (w339:string)
          }
        }
        n227 = Format Date/Time String(time format string (%c)="%m/%d/%Y", seconds (now)=w290, UTC format=FALSE) -> (date/time string=w289:string)
        n228 = Format Date/Time String(time format string (%c)="%H:%M:%S%4u", seconds (now)=w293, UTC format=FALSE) -> (date/time string=w288:string)
        n229 = Build Array(w289) -> (w287:string[])
        n230 = Build Array(w288) -> (w286:string[])
        n231 = Build Array(w275) -> (w274:string[])
        n232 = call <instrlib>:"Configure Current Output.vi"("VISA resource name"=w330, "Current Immediate Amplitude (0 A)"=0.0, "error in (no error)"=w329) -> ("VISA resource name out"=w310:refnum<visa-resource-name>, "error out"=w311:errorcluster)  [unwired: 11 in]
        n233 = Build Array(w276) -> (w285:dbl[])
        n234 = Build Array(w280) -> (w283:dbl[])
        n235 = Number To Engineering String(4:w285) -> (0:w281:string[])  [unwired: 3 in]
        n236 = Number To Engineering String(4:w283) -> (0:w282:string[])  [unwired: 3 in]
        n237 = Build Array(w287, w286, w274, w281, w282) -> (w284:string[][])
        n238 = TDMS Write(0:w268, 5:"Aggregated Data" ("group name"), 7:string[] ["Date", "Time", "Run Number", "Ic (A)", "n value"] ("channel name(s) in (Untitled)"), 9:w284, 11:w267) -> (4:w272:refnum<k34>, 15:w273:errorcluster)  [unwired: 1 in, 2 out]
      }
      "Errors?" <- w115
      n239 = call <instrlib>:"Close.vi"("error in (no error)"=w148, "VISA resource name"=w147) -> ("error out"=w149:errorcluster)  [unwired: 9 in]
      n240 = TDMS Close(8:w132, 11:w125) -> (0:w140:errorcluster)  [unwired: 1 out]
      n241 = call <instrlib>:"Close.vi"("error in (no error)"=w145, "VISA resource name"=w144) -> ("error out"=w146:errorcluster)  [unwired: 9 in]
      n242 = call <vilib>:"Simple Error Handler.vi"("error in (no error)"=w140) -> ()  [unwired: 2 in, 7 out]
      n243 = call <vilib>:"Simple Error Handler.vi"("error in (no error)"=w149) -> ()  [unwired: 4 in, 5 out]
      n244 = call <vilib>:"Simple Error Handler.vi"("error in (no error)"=w146) -> ()  [unwired: 4 in, 5 out]
    }
  }
